vi "SetupDAQ.vi"(0 "number of samples":i32=1000, 1 "rate":dbl=1000.0, 3 "input terminal configuration":i32(ring)=10083 items=["default"=-1, "RSE"=10083, "NRSE"=10078, "Differential"=10106, "Pseudodifferential"=12529], 4 "input terminal configuration 2":i32(ring)=10083 items=["default"=-1, "RSE"=10083, "NRSE"=10078, "Differential"=10106, "Pseudodifferential"=12529], 5 "error in":errorcluster, 6 "physical channel":string="Dev2/ai0", 8 "physical channel 2":string="Dev2/ai1", 10 "physical channel 3":string="Dev2/ai0", 12 "physical channel 4":string="Dev2/ai0") -> (14 "task out":refnum<k21>, 19 "error out":errorcluster)   [LabVIEW 2017]
uses:
  <vilib>/DAQmx/configure/timing.llb/DAQmx Timing (Sample Clock).vi
  <vilib>/DAQmx/create/channels.llb/DAQmx Create Channel (AI-Voltage-Basic).vi
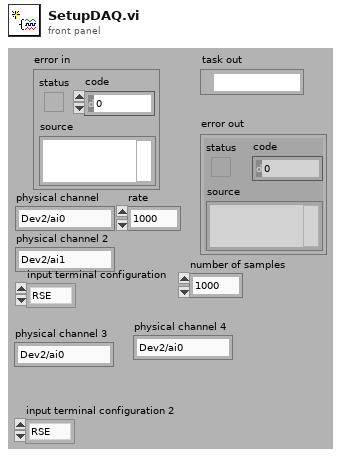
[diagram p1: front panel]
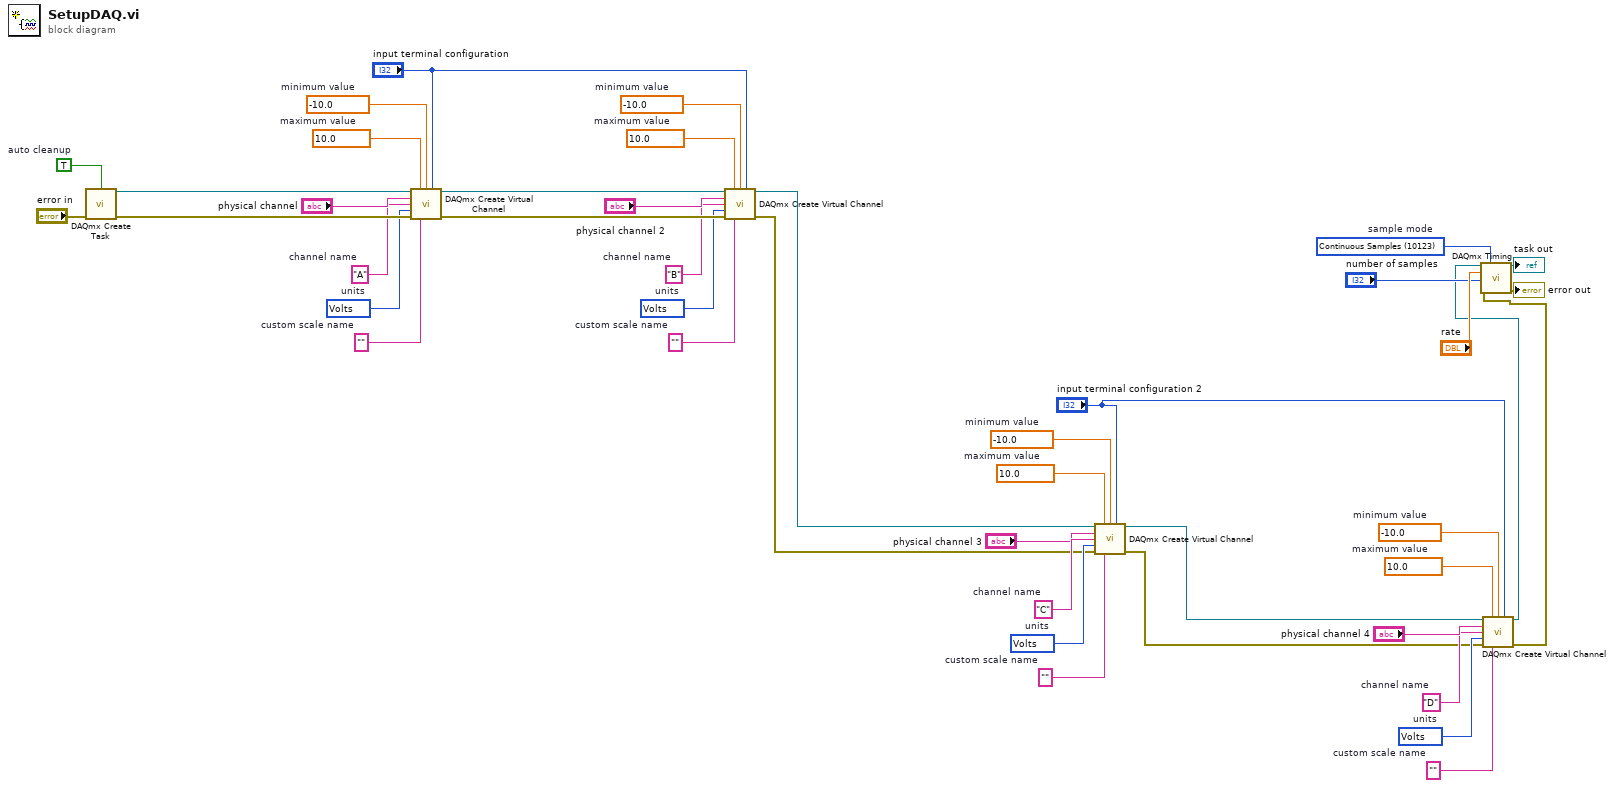
[diagram p0: block diagram]
diagram:
  w8 = 10348 items=["Volts"=10348, "From Custom Scale"=10065]  # units
  w9 = "D"  # channel name
  w10 = ""  # custom scale name
  w11 = -10.0  # minimum value
  w12 = 10.0  # maximum value
  w19 = 10348 items=["Volts"=10348, "From Custom Scale"=10065]  # units
  w18 = "C"  # channel name
  w17 = ""  # custom scale name
  w16 = -10.0  # minimum value
  w15 = 10.0  # maximum value
  w21 = 10123 items=["Finite Samples"=10178, "Continuous Samples"=10123, "Hardware Timed Single Point"=12522]  # sample mode
  w26 = 10348 items=["Volts"=10348, "From Custom Scale"=10065]  # units
  w27 = "B"  # channel name
  w28 = ""  # custom scale name
  w29 = -10.0  # minimum value
  w30 = 10.0  # maximum value
  w33 = 10348 items=["Volts"=10348, "From Custom Scale"=10065]  # units
  w34 = "A"  # channel name
  w36 = ""  # custom scale name
  w37 = -10.0  # minimum value
  w38 = 10.0  # maximum value
  w41 = TRUE  # auto cleanup
  n1 = call <vilib>:"DAQmx Create Task.vi"("auto cleanup"=w41, "error in"="error in") -> ("task out"=w40:refnum<k21>, "error out"=w42:errorcluster)  [unwired: 3 in, 9 out]
  n2 = call-poly <vilib>:"DAQmx Create Virtual Channel.vi"("task in"=w40, "maximum value"=w38, "minimum value"=w37, "input terminal configuration"="input terminal configuration", "physical channels"="physical channel", "name to assign"=w34, "units"=w33, "error in"=w42, "custom scale name"=w36) -> ("task out"=w32:refnum<k21>, "error out"=w35:errorcluster)  [unwired: 5 out]
  n3 = call-poly <vilib>:"DAQmx Create Virtual Channel.vi"("task in"=w32, "maximum value"=w30, "minimum value"=w29, "input terminal configuration"="input terminal configuration", "physical channels"="physical channel 2", "name to assign"=w27, "units"=w26, "error in"=w35, "custom scale name"=w28) -> ("task out"=w7:refnum<k21>, "error out"=w6:errorcluster)  [unwired: 5 out]
  n4 = call-poly <vilib>:"DAQmx Create Virtual Channel.vi"("task in"=w7, "maximum value"=w15, "minimum value"=w16, "input terminal configuration"="input terminal configuration 2", "physical channels"="physical channel 3", "name to assign"=w18, "units"=w19, "error in"=w6, "custom scale name"=w17) -> ("task out"=w5:refnum<k21>, "error out"=w4:errorcluster)  [unwired: 5 out]
  n5 = call-poly <vilib>:"DAQmx Create Virtual Channel.vi"("task in"=w5, "maximum value"=w12, "minimum value"=w11, "input terminal configuration"="input terminal configuration 2", "physical channels"="physical channel 4", "name to assign"=w9, "units"=w8, "error in"=w4, "custom scale name"=w10) -> ("task out"=w2:refnum<k21>, "error out"=w1:errorcluster)  [unwired: 5 out]
  n6 = call-poly <vilib>:"DAQmx Timing.vi"("task/channels in"=w2, "sample mode"=w21, "samples per channel"="number of samples", "rate"="rate", "error in"=w1) -> ("task out"=→"task out":refnum<k21>, "error out"=→"error out":errorcluster)  [unwired: 2 in, 7 out]
